vi "MC - Test Key Names.vi"(1 "index":i32, 2 "Key Name":string[][](array[string])) -> (0 "key name valid":bool)   [LabVIEW 2015]
panel:
  in  "Enum":T1(ring)
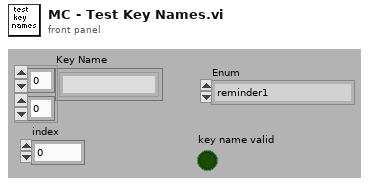
[diagram p1: front panel]
types:
  T1 = enum16{"reminder1", "reminder2", "reminder3", "reminder4", "reminder5", "reminder6", "reminder7", "reminder8", "reminder9", "reminder10"}
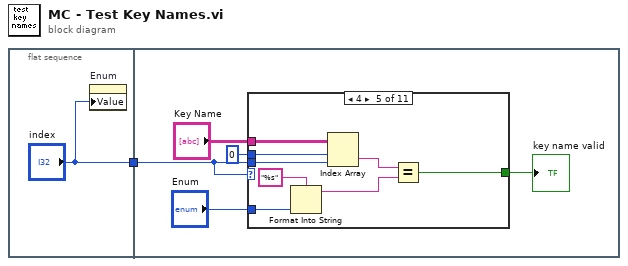
[diagram p0: block diagram]
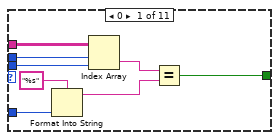
[diagram p2: hidden frame]
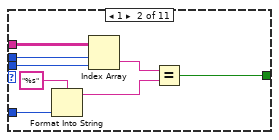
[diagram p3: hidden frame]
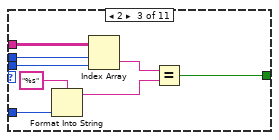
[diagram p4: hidden frame]
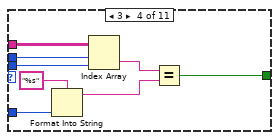
[diagram p5: hidden frame]
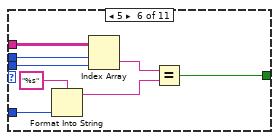
[diagram p6: hidden frame]
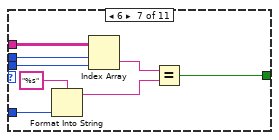
[diagram p7: hidden frame]
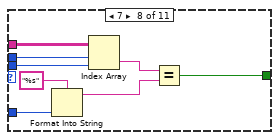
[diagram p8: hidden frame]
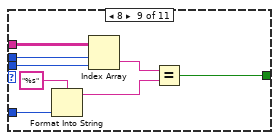
[diagram p9: hidden frame]
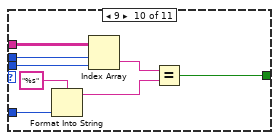
[diagram p10: hidden frame]
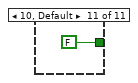
[diagram p11: hidden frame]
diagram:
  n1 = flat-sequence {
    tunnel: ["index"] -> w1
    tunnel: w1 -> [w4]
    frame #0 {
      n2 = property on="Enum" class="Enum (strict)"("Value"="index") -> ()  [unwired: 2 in, 2 out]
    }
    frame #1 {
      n3 = case shown="4" w4 {
        tunnel: w4 -> [w14 w22 w30 w38 w46 w54 w62 w70 w78 w86 _]
        tunnel: 0 ("Index") -> [w15 w23 w31 w39 w47 w55 w63 w71 w79 w87 _]
        tunnel: "Key Name" -> [w13 w21 w29 w37 w45 w53 w61 w69 w77 w85 _]
        tunnel: [w11 w19 w27 w35 w43 w51 w59 w67 w75 w83 FALSE] -> w3
        tunnel: "Enum" -> [w10 w18 w26 w34 w42 w50 w58 w66 w74 w82 _]
        frame 0 {
          n4 = Format Into String(format string="%s", w10) -> (resulting string=w8:string)  [unwired: 2 in, 1 out]
          n5 = Index Array(array=w13, index (row)=w15, index (col)=w14) -> (element=w12:string)
          n6 = Equal?(x=w12, y=w8) -> (x = y?=w11:bool)
        }
        frame 1 {
          n7 = Format Into String(format string="%s", w18) -> (resulting string=w16:string)  [unwired: 2 in, 1 out]
          n8 = Index Array(array=w21, index (row)=w23, index (col)=w22) -> (element=w20:string)
          n9 = Equal?(x=w20, y=w16) -> (x = y?=w19:bool)
        }
        frame 2 {
          n10 = Format Into String(format string="%s", w26) -> (resulting string=w24:string)  [unwired: 2 in, 1 out]
          n11 = Index Array(array=w29, index (row)=w31, index (col)=w30) -> (element=w28:string)
          n12 = Equal?(x=w28, y=w24) -> (x = y?=w27:bool)
        }
        frame 3 {
          n13 = Format Into String(format string="%s", w34) -> (resulting string=w32:string)  [unwired: 2 in, 1 out]
          n14 = Index Array(array=w37, index (row)=w39, index (col)=w38) -> (element=w36:string)
          n15 = Equal?(x=w36, y=w32) -> (x = y?=w35:bool)
        }
        frame 4 {
          n16 = Format Into String(format string="%s", w42) -> (resulting string=w40:string)  [unwired: 2 in, 1 out]
          n17 = Index Array(array=w45, index (row)=w47, index (col)=w46) -> (element=w44:string)
          n18 = Equal?(x=w44, y=w40) -> (x = y?=w43:bool)
        }
        frame 5 {
          n19 = Format Into String(format string="%s", w50) -> (resulting string=w48:string)  [unwired: 2 in, 1 out]
          n20 = Index Array(array=w53, index (row)=w55, index (col)=w54) -> (element=w52:string)
          n21 = Equal?(x=w52, y=w48) -> (x = y?=w51:bool)
        }
        frame 6 {
          n22 = Format Into String(format string="%s", w58) -> (resulting string=w56:string)  [unwired: 2 in, 1 out]
          n23 = Index Array(array=w61, index (row)=w63, index (col)=w62) -> (element=w60:string)
          n24 = Equal?(x=w60, y=w56) -> (x = y?=w59:bool)
        }
        frame 7 {
          n25 = Format Into String(format string="%s", w66) -> (resulting string=w64:string)  [unwired: 2 in, 1 out]
          n26 = Index Array(array=w69, index (row)=w71, index (col)=w70) -> (element=w68:string)
          n27 = Equal?(x=w68, y=w64) -> (x = y?=w67:bool)
        }
        frame 8 {
          n28 = Format Into String(format string="%s", w74) -> (resulting string=w72:string)  [unwired: 2 in, 1 out]
          n29 = Index Array(array=w77, index (row)=w79, index (col)=w78) -> (element=w76:string)
          n30 = Equal?(x=w76, y=w72) -> (x = y?=w75:bool)
        }
        frame 9 {
          n31 = Format Into String(format string="%s", w82) -> (resulting string=w80:string)  [unwired: 2 in, 1 out]
          n32 = Index Array(array=w85, index (row)=w87, index (col)=w86) -> (element=w84:string)
          n33 = Equal?(x=w84, y=w80) -> (x = y?=w83:bool)
        }
        frame 10, Default {
        }
      }
      "key name valid" <- w3
    }
  }
